vi "OSC Waveform.vi"(1 "Sampling information":cluster{"Fs":dbl, "#s":dbl}[](array[cluster])=[{"Fs"=200000.00004074536, "#s"=20000.0}], 2 "OSC Configuration":T1(array[cluster])=[{"Signal Type"=enum."Sine Wave", "DC"=0.0, "Amplitude"=0.2, "frequency"=20.0, "Phase"=0.0}] {"frequency" format="%0.2p"; "Amplitude" format="%0.2p"; "DC" format="%.2p"}) -> (0 "OSC Waveforms":waveform(dbl)[][](array[waveform]))   [LabVIEW 2011]
uses:
  <vilib>/measure/NI_MABase.lvlib
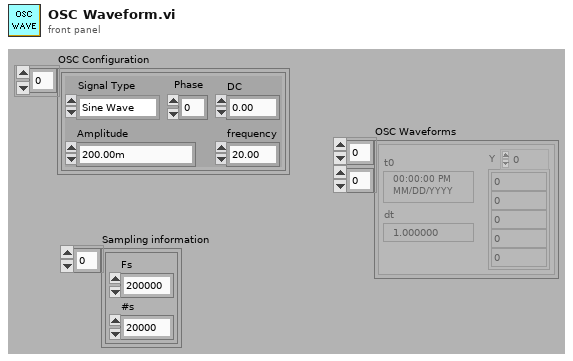
[diagram p1: front panel]
types:
  T1 = cluster{"Signal Type":enum16{"Sine Wave", "Triangle Wave", "Square Wave", "Sawtooth Wave"}, "DC":dbl, "Amplitude":dbl, "frequency":dbl, "Phase":dbl}[]
  T2 = enum16{"Sine Wave", "Triangle Wave", "Square Wave", "Sawtooth Wave"}
  T3 = cluster{"Signal Type":enum16{"Sine Wave", "Triangle Wave", "Square Wave", "Sawtooth Wave"}, "DC":dbl, "Amplitude":dbl, "frequency":dbl, "Phase":dbl}
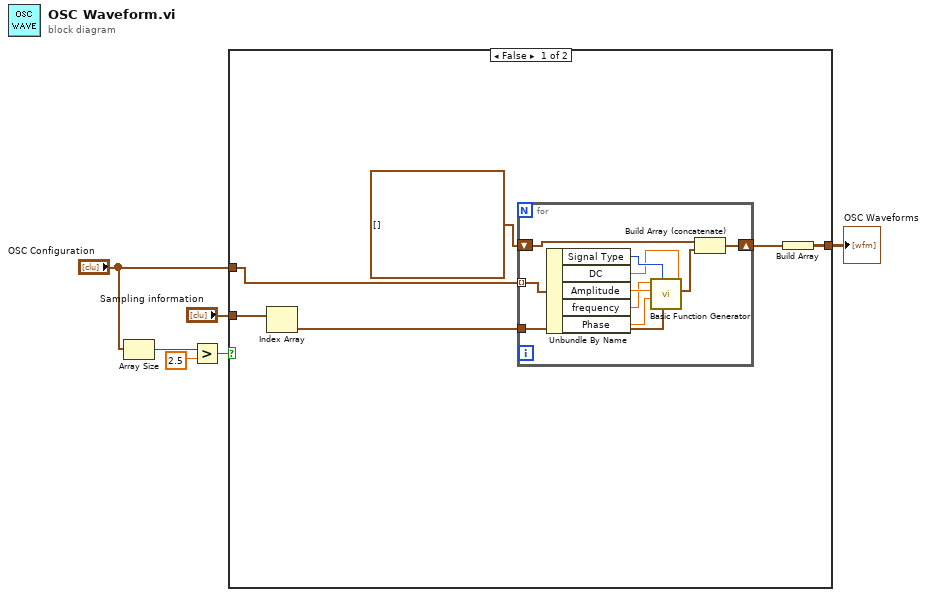
[diagram p0: block diagram]
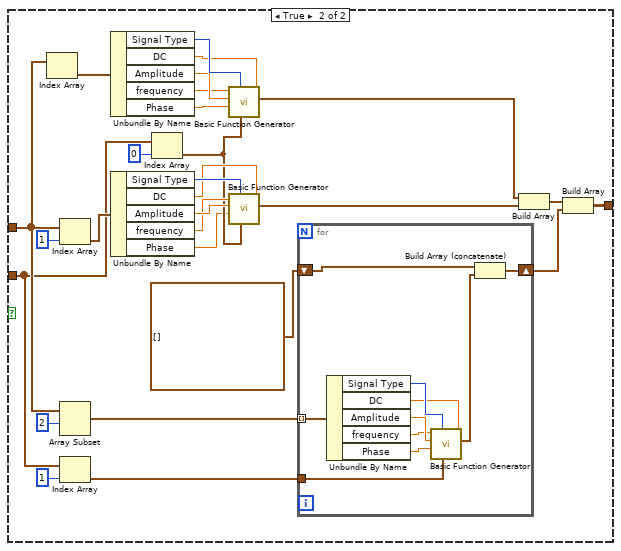
[diagram p2: hidden frame]
diagram:
  n1 = Array Size(array="OSC Configuration") -> (size(s)=w4:i32)
  n2 = Greater?(x=w4, y=2.5) -> (0:w2:bool)
  n3 = case shown="False" w2 {
    tunnel: "OSC Configuration" -> [w12 w37]
    tunnel: [w10 w34] -> w1
    tunnel: "Sampling information" -> [w8 w27]
    frame False {
      n4 = Index Array(array=w8) -> (element=w7:cluster{"Fs":dbl, "#s":dbl})  [unwired: 1 in]
      n5 = for {
        tunnel: w12 -> [w22] mode=indexing
        shift-right: [w17] -> w11
        shift-left: waveform(dbl)[] [] -> [w15]
        tunnel: w7 -> [w16]
        n6 = Unbundle By Name(w22) -> ("Signal Type"=w21:T2, "DC"=w20:dbl, "Amplitude"=w19:dbl, "frequency"=w18:dbl, "Phase"=w13:dbl)
        n7 = call <vilib>:"Basic Function Generator.vi"("offset"=w20, "sampling info"=w16, "signal type"=w21, "phase"=w13, "amplitude"=w19, "frequency"=w18) -> ("signal out"=w14:waveform(dbl))  [unwired: 3 in, 2 out]
        n8 = Build Array (concatenate)(w15, w14) -> (w17:waveform(dbl)[])
      }
      n9 = Build Array(w11) -> (w10:waveform(dbl)[][])
    }
    frame True {
      n10 = Index Array(array=w37) -> (element=w48:T3)  [unwired: 1 in]
      n11 = Index Array(array=w37, index=1) -> (element=w47:T3)
      n12 = Array Subset(array=w37, index=2) -> (w35:T1)  [unwired: 1 in]
      n13 = Index Array(array=w27, index=1) -> (element=w26:cluster{"Fs":dbl, "#s":dbl})
      n14 = Unbundle By Name(w48) -> ("Signal Type"=w46:T2, "DC"=w45:dbl, "Amplitude"=w44:dbl, "frequency"=w43:dbl, "Phase"=w24:dbl)
      n15 = Unbundle By Name(w47) -> ("Signal Type"=w42:T2, "DC"=w41:dbl, "Amplitude"=w40:dbl, "frequency"=w39:dbl, "Phase"=w23:dbl)
      n16 = Index Array(array=w27, index=0) -> (element=w28:cluster{"Fs":dbl, "#s":dbl})
      n17 = call <vilib>:"Basic Function Generator.vi"("offset"=w45, "sampling info"=w28, "signal type"=w46, "phase"=w24, "amplitude"=w44, "frequency"=w43) -> ("signal out"=w25:waveform(dbl))  [unwired: 3 in, 2 out]
      n18 = call <vilib>:"Basic Function Generator.vi"("offset"=w41, "sampling info"=w28, "signal type"=w42, "phase"=w23, "amplitude"=w40, "frequency"=w39) -> ("signal out"=w38:waveform(dbl))  [unwired: 3 in, 2 out]
      n19 = for {
        tunnel: w35 -> [w59] mode=indexing
        shift-right: [w54] -> w32
        shift-left: waveform(dbl)[] [] -> [w51]
        tunnel: w26 -> [w53]
        n20 = Unbundle By Name(w59) -> ("Signal Type"=w58:T2, "DC"=w57:dbl, "Amplitude"=w56:dbl, "frequency"=w55:dbl, "Phase"=w50:dbl)
        n21 = call <vilib>:"Basic Function Generator.vi"("offset"=w57, "sampling info"=w53, "signal type"=w58, "phase"=w50, "amplitude"=w56, "frequency"=w55) -> ("signal out"=w52:waveform(dbl))  [unwired: 3 in, 2 out]
        n22 = Build Array (concatenate)(w51, w52) -> (w54:waveform(dbl)[])
      }
      n23 = Build Array(w25, w38) -> (w31:waveform(dbl)[])
      n24 = Build Array(w31, w32) -> (w34:waveform(dbl)[][])
    }
  }
  "OSC Waveforms" <- w1
